vi "test_image_avg.vi"() -> ()   [LabVIEW 2013]
panel:
  out "Numeric":i32
  in  "stop":bool
  out "output array":dbl[][](array[numeric])
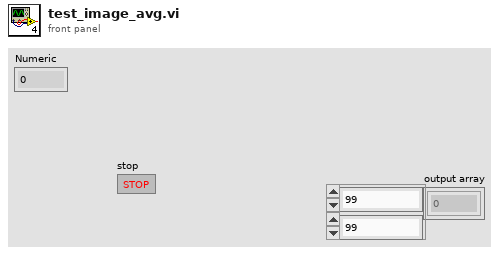
[diagram p1: front panel]
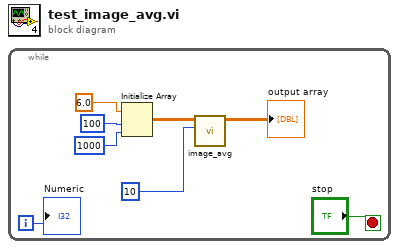
[diagram p0: block diagram]
diagram:
  n1 = while {
    i -> [w1]
    stop <- "stop" stop-if-true
    n2 = Initialize Array(6.0 ("element"), 100 ("dimension size"), 1000 ("dimension size")) -> (w4:dbl[][])
    n3 = call "image_avg.vi"("points / pixel"=10, "input array"=w4) -> ("output array"=→"output array":dbl[][])  [unwired: 9 in]
    "Numeric" <- w1
  }
